vi "MVE Security.vi"(10 "Item Path":string, 11 "ACL In":string) -> (3 "ACL Out":string)   [LabVIEW 2016]
uses:
  <vilib>/Platform/security/user/NI_Security Privilege Descriptor.ctl
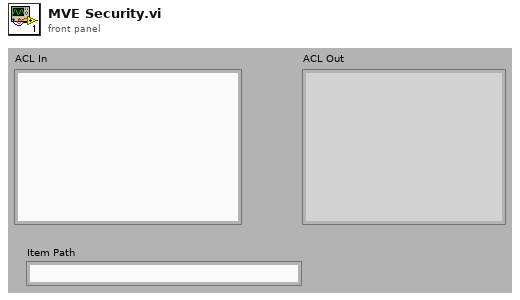
[diagram p1: front panel]
types:
  T1 = typedef "NI_Security Privilege Descriptor.ctl" = cluster{"Privilege Name":string, "Privilege ID":u32}
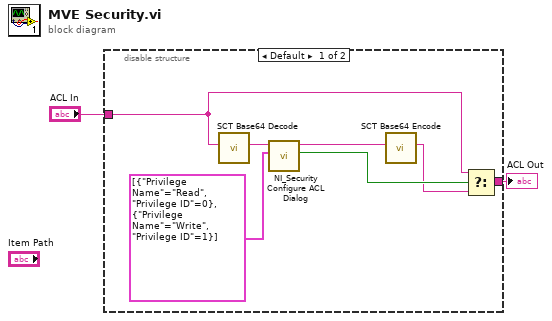
[diagram p0: block diagram]
diagram:
  n1 = disable-structure shown="Default" {
    disable-tunnel: [w5 w10] -> w2
    disable-tunnel: "ACL In" -> [w4 w10]
    frame condition #0 (active) {
      n2 = call <resource>:"SCT Base64 Decode.vi"("buffer in"=w4) -> ("base64 decoded buffer"=w8:string)  [unwired: 9 in, 1 out]
      n3 = call <vilib>:"NI_Security Configure ACL Dialog.vi"("privileges"=T1[] [{"Privilege Name"="Read", "Privilege ID"=0}, {"Privilege Name"="Write", "Privilege ID"=1}], "ACL In"=w8) -> ("Cancelled"=w7:bool, "ACL Out"=w9:string)  [unwired: 7 in, 1 out]
      n4 = call <resource>:"SCT Base64 Encode.vi"("buffer in"=w9) -> ("base64 encoded buffer"=w6:string)  [unwired: 10 in]
      n5 = Select(t=w4, s=w7, f=w6) -> (s? t:f=w5:string)
    }
    frame condition #1 {
    }
  }
  "ACL Out" <- w2
